vi "Get Picture.vi"(8 "error in (no error)":errorcluster, 11 "Logic Circuit in":refnum<class "Logic Circuit.lvclass">) -> (0 "error out":errorcluster, 2 "Picture":picture, 3 "Logic Circuit out":refnum<class "Logic Circuit.lvclass">)   [LabVIEW 2020, in "Logic Circuit.lvclass"]
uses:
  Logic Circuit.lvclass
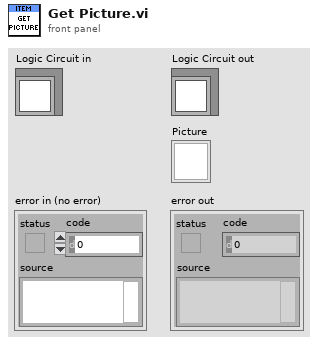
[diagram p1: front panel]
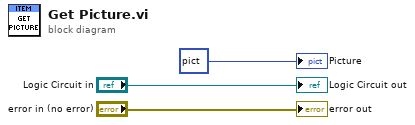
[diagram p0: block diagram]
diagram:
  "error out" <- "error in (no error)"
  "Logic Circuit out" <- "Logic Circuit in"
  "Picture" <- picture bytes[3230] ("new picture")
